vi "Word Example.vi"() -> ()   [LabVIEW 2017]
uses:
  LabVIEW NPOI/MS-Word/MS-Word.lvclass
  C:/Users/Neo/Desktop/Dev_Tools_BR/LabVIEW_NPOI/src/LabVIEW NPOI/Document/Document.lvclass
  LabVIEW NPOI/Document/Document.lvclass/Document.ctl
  LabVIEW NPOI/Document/Get FilePath.vi
  LabVIEW NPOI/Document/Append Table (double).vi
  LabVIEW NPOI/Document/Append Table (string).vi
  LabVIEW NPOI/Document/Read Table As String.vi
  LabVIEW NPOI/Document/Document.lvclass
panel:
  in  "createDocumentBttn":bool
  in  "Text":string="Lorem ipsum dolor sit amet, consectetur adipiscing elit, sed do eiusmod tempor incididunt ut labore et dolore magna aliqua. Adipiscing bibendum est ultricies integer quis auctor elit sed vulputate. Volutpat consequat mauris nunc congue nisi vitae suscipit tellus. Eget arcu dictum varius duis at consectetur lorem donec massa. Morbi enim nunc faucibus a pellentesque sit. Risus ultricies tristique nulla aliquet enim tortor at. Sit amet consectetur adipiscing elit ut aliquam purus sit. Porta lorem mollis aliquam ut porttitor leo a diam. Odio aenean sed adipiscing diam donec adipiscing tristique risus. Nunc eget lorem dolor sed viverra ipsum nunc aliquet. Ultrices gravida dictum fusce ut. Mi eget mauris pharetra et ultrices. Ultrices dui sapien eget mi proin. Duis ut diam quam nulla porttitor massa id neque. Eu lobortis elementum nibh tellus molestie nunc non. Iaculis nunc sed augue lacus viverra. Enim sed faucibus turpis in eu. Quis viverra nibh cras pulvinar mattis. Auctor augue mauris augue neque gravida. Enim ut tellus elementum sagittis vitae."
  in  "addParagraphBttn":bool
  in  "HTML File Path":path
  in  "convertToHtml":bool
  out "Read Table Time":u32
  out "Add Table Time":u32
  in  "addImageBttn":bool
  out "Table Control":string[][](table)
  in  "readTableBttn":bool
  in  "#Columns":i32=100
  in  "#Rows":i32=2
  in  "tableType":enum32{"Strings", "Doubles"}(radio)
  in  "addTableBttn":bool
  out "FilePath":path
  in  "openDocumentBttn":bool
  in  "baseDocumentPath":path caption="Folder Path"
  in  "saveAsDocumentBttn":bool
  in  "saveDocumentBttn":bool
  in  "documentName":string="Book1.xlsx" caption="Name"
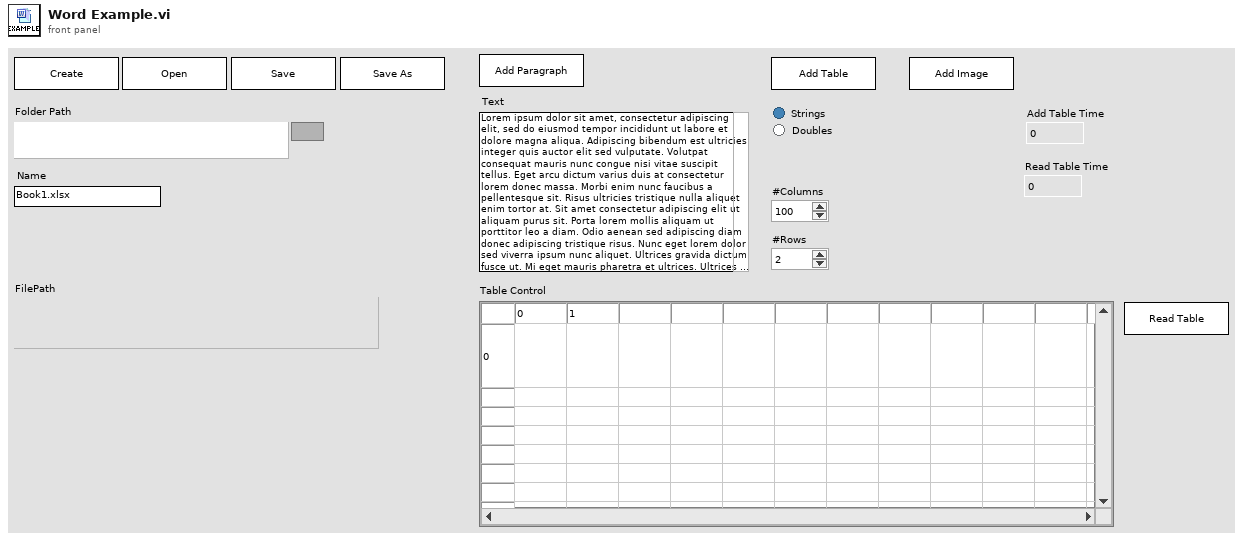
[diagram p1: front panel]
types:
  T1 = cluster{"documentObject":refnum<class "MS-Word.lvclass">, "documentPath":path, "documentName":string, "pageName":string, "styleName":string, "ctlRefs":refnum<vi>[]}
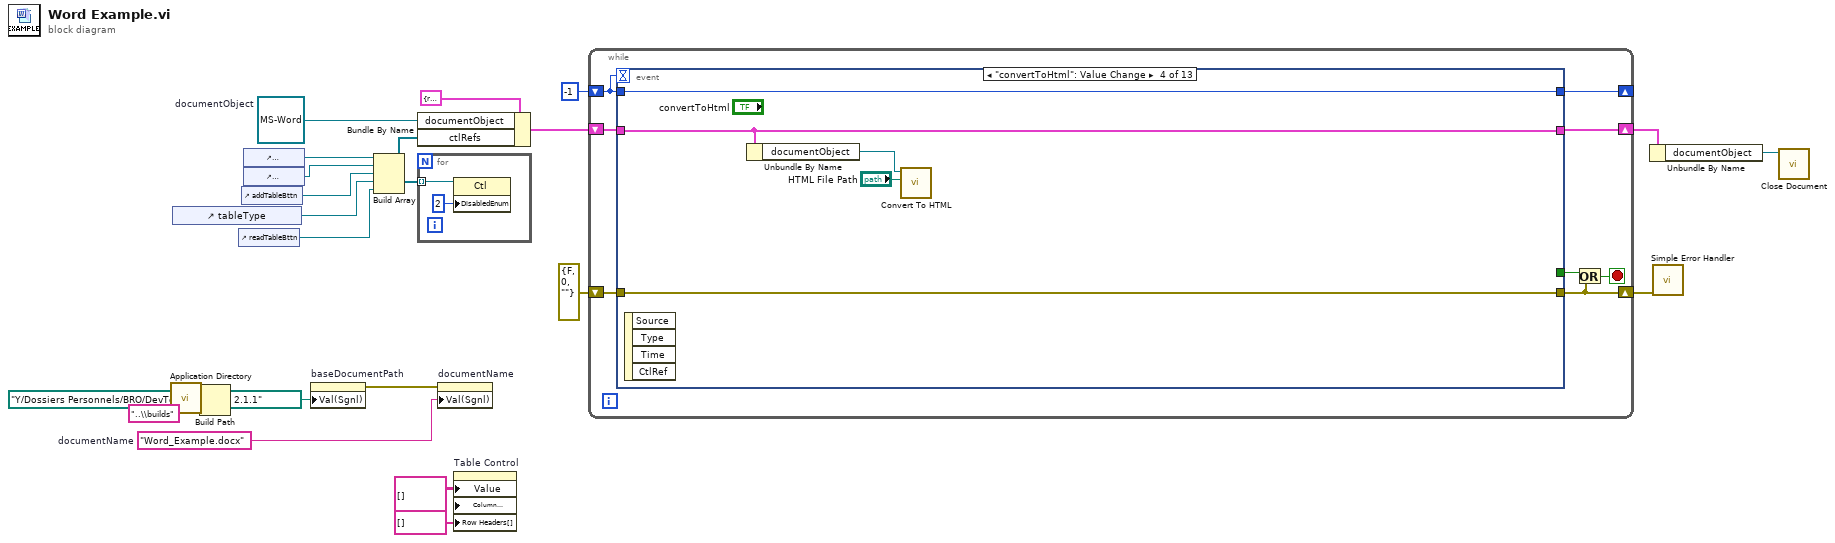
[diagram p0: block diagram]
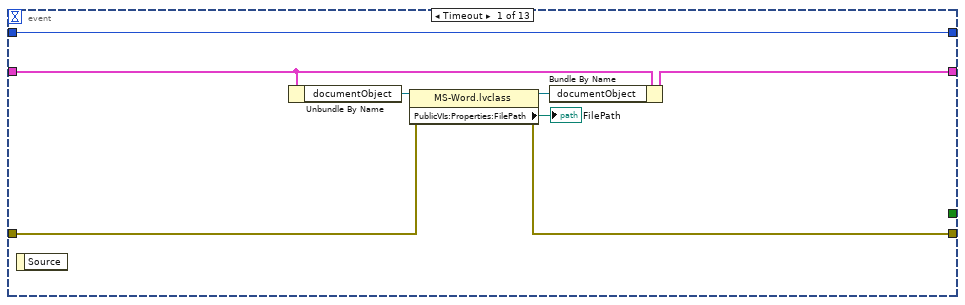
[diagram p2: hidden frame]
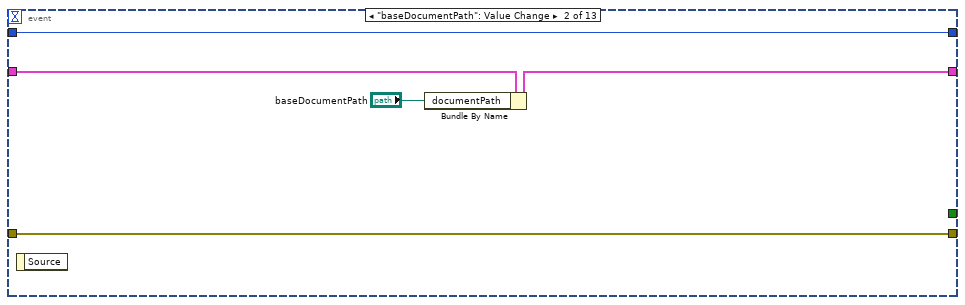
[diagram p3: hidden frame]
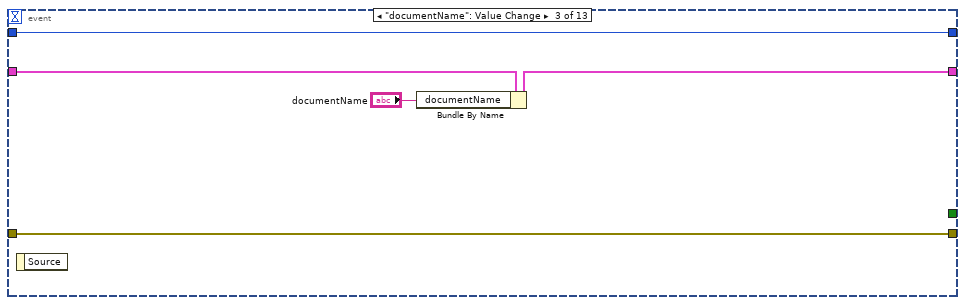
[diagram p4: hidden frame]
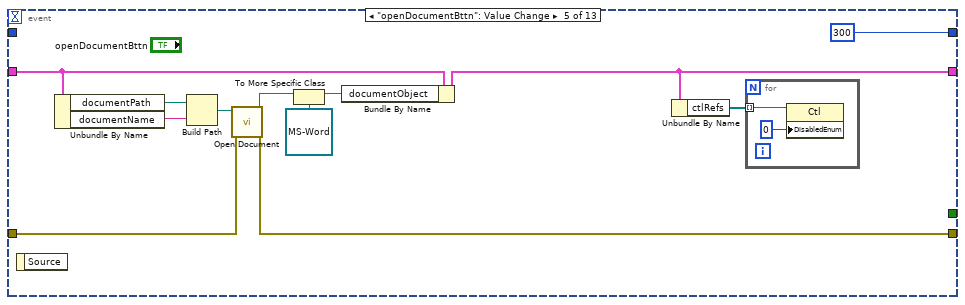
[diagram p5: hidden frame]
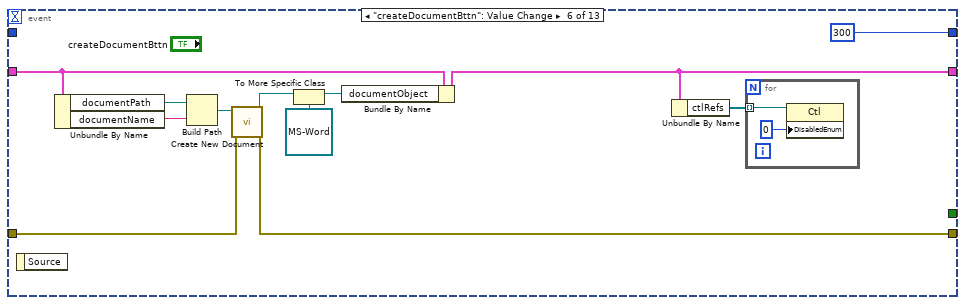
[diagram p6: hidden frame]
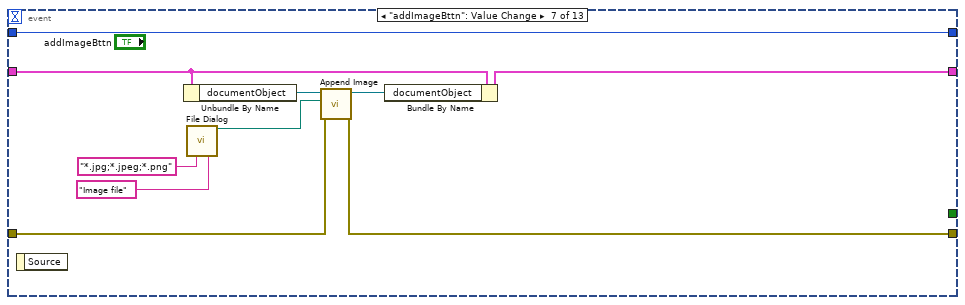
[diagram p7: hidden frame]
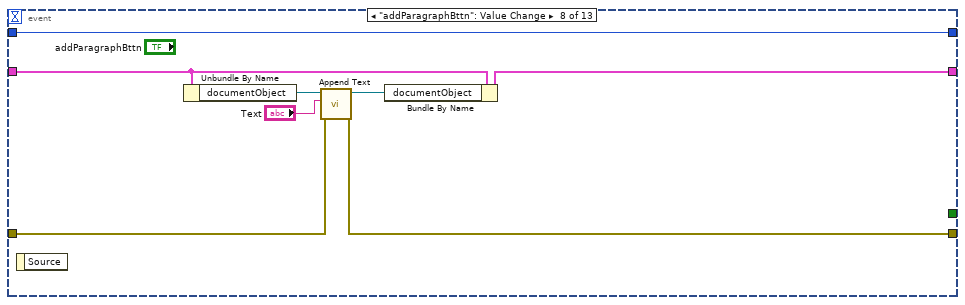
[diagram p8: hidden frame]
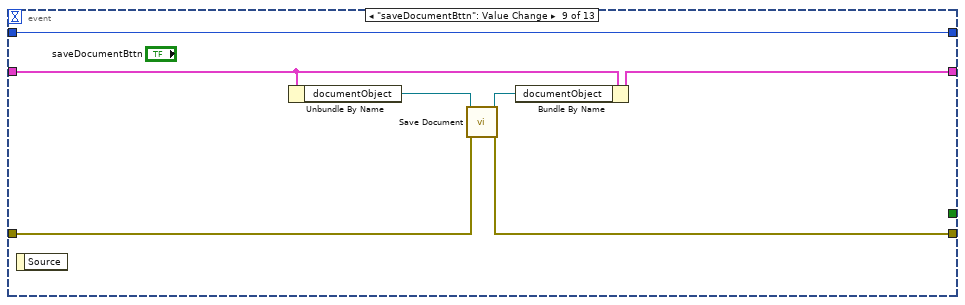
[diagram p9: hidden frame]
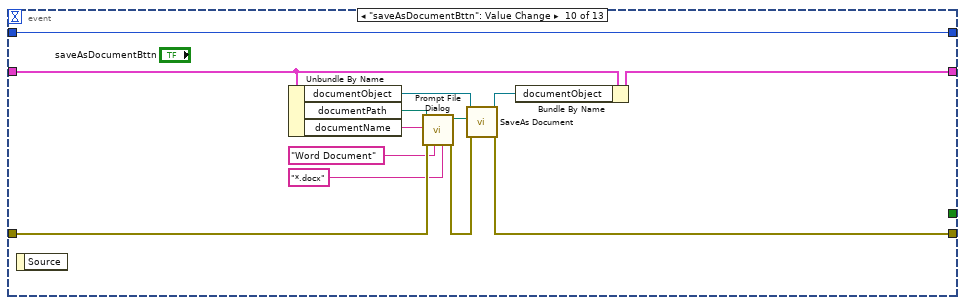
[diagram p10: hidden frame]
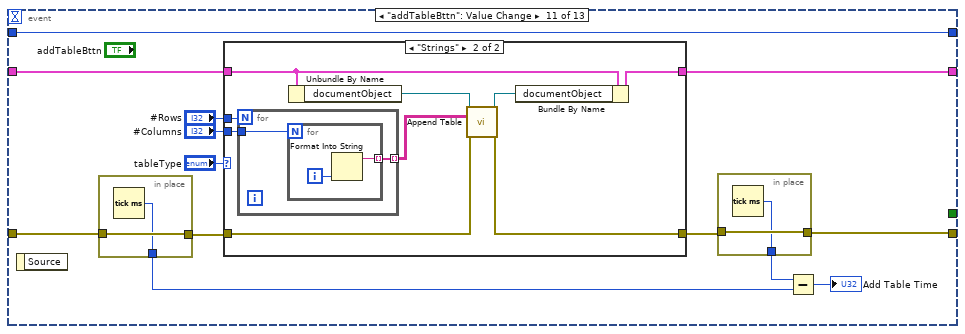
[diagram p11: hidden frame]
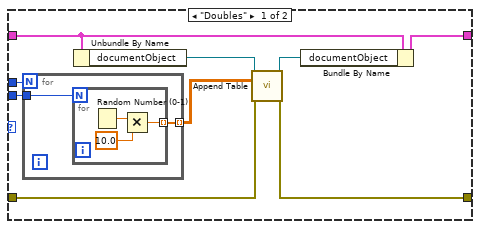
[diagram p12: hidden frame]
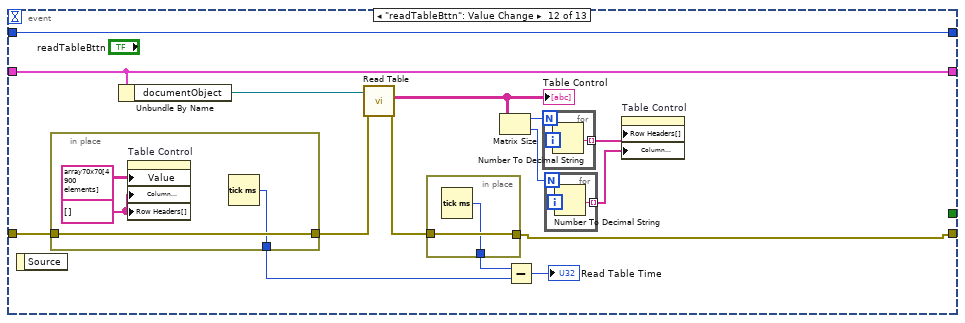
[diagram p13: hidden frame]
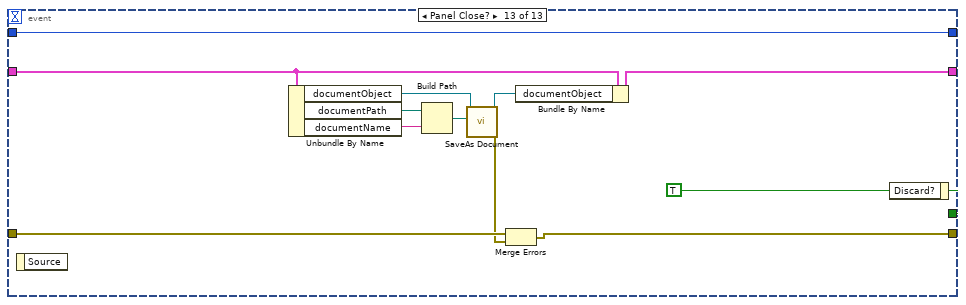
[diagram p14: hidden frame]
diagram:
  w5 = string[] [] ("Row Header Strings[]")
  w10 = "Word_Example.docx"  # documentName
  w14 = refnum<class "MS-Word.lvclass"> refnum  # documentObject
  n1 = call <vilib>:"Application Directory.vi"() -> ("Application Directory"=w4:path)
  n2 = control-ref of="tableType"() -> (w8:refnum<vi>)
  n3 = Build Path(base path=w4, name or relative path="..\\builds") -> ()  [unwired: 1 out]
  n4 = control-ref of="readTableBttn"() -> (w7:refnum<vi>)
  n5 = control-ref of="addTableBttn"() -> (w9:refnum<vi>)
  n6 = control-ref of="saveDocumentBttn"() -> (w13:refnum<vi>)
  n7 = control-ref of="saveAsDocumentBttn"() -> (w12:refnum<vi>)
  n8 = property on="baseDocumentPath" class="Path"("Val(Sgnl)"=path "Y:/Dossiers Personnels/BRO/DevTools_BR/NPOI 2.1.1" ("Value (Signaling)")) -> (error out=w2:errorcluster)  [unwired: 2 in, 1 out]
  n9 = Build Array(w13, w12, w9, w8, w7) -> (w11:refnum<vi>[])
  n10 = Bundle By Name(cluster=T1 {"documentObject"=refnum, "documentPath"=path "", "documentName"="", "pageName"="", "styleName"="Default", "ctlRefs"=[]}, "documentObject"=w14, "ctlRefs"=w11) -> (w21:T1)
  n11 = for {
    tunnel: w11 -> [w23] mode=indexing
    n12 = property class="Ctl"(reference=w23, "DisabledEnum"=u8 2) -> ()  [unwired: 1 in, 2 out]
  }
  n13 = property on="documentName" class="Str"(error in=w2, "Val(Sgnl)"=w10) -> ()  [unwired: 1 in, 2 out]
  n14 = property on="Table Control" class="Tbl (strict)"("Value"=string[][] [] ("Table Control"), "Column Headers[]"=w5, "Row Headers[]"=w5) -> ()  [unwired: 2 in, 2 out]
  n15 = while {
    shift-right: [w30] -> w17
    shift-left: w21 -> [w31]
    shift-right: [w28] -> w20
    shift-left: errorcluster {"status"=FALSE, "code"=0, "source"=""} ("error IO") -> [w29]
    shift-right: [w24] -> _
    shift-left: -1 -> [w25]
    stop <- w26 stop-if-true
    n16 = event shown="[3] \"convertToHtml\": Value Change" {
      selector: _ -> [_ _ _ _ _ _ _ _ _ _ _ _ _]
      dyn-events: _ -> [_ _ _ _ _ _ _ _ _ _ _ _ _]
      timeout: w25 -> [_ _ _ _ _ _ _ _ _ _ _ _ _]
      tunnel: [_ _ _ _ _ _ _ _ _ _ _ _ w194] -> w27
      tunnel: w31 -> [w39 w44 w49 w52 w66 w80 w91 w99 w107 w120 w128 w178 w201]
      tunnel: [w32 w43 w48 w52 w61 w75 w87 w95 w105 w118 w133 w178 w196] -> w30
      tunnel: [w35 w41 w46 w54 w55 w69 w88 w96 w103 w116 w124 w168 w192] -> w28
      tunnel: w29 -> [w36 w41 w46 w54 w63 w77 w89 w97 w102 w114 w127 w171 w193]
      tunnel: w25 -> [w33 w40 w45 w53 _ _ w92 w100 w101 w108 w132 w179 w190]
      tunnel: [w33 w40 w45 w53 300 300 w92 w100 w101 w108 w132 w179 w190] -> w24
      event Timeout {
        n17 = event-data() -> ()  [unwired: 1 in, 1 out]
        n18 = Unbundle By Name(w39) -> ("documentObject"=w38:refnum<class "MS-Word.lvclass">)
        n19 = property class="MS-Word.lvclass"(reference=w38, error in=w36) -> (reference out=w37:refnum<class "MS-Word.lvclass">, error out=w35:errorcluster, "PublicVIs:Properties:FilePath"=→"FilePath":path)
        n20 = Bundle By Name(cluster=w39, "documentObject"=w37) -> (w32:T1)
      }
      event "baseDocumentPath": Value Change {
        n21 = event-data() -> ()  [unwired: 1 in, 1 out]
        n22 = Bundle By Name(cluster=w44, "documentPath"="baseDocumentPath") -> (w43:T1)
      }
      event "documentName": Value Change {
        n23 = event-data() -> ()  [unwired: 1 in, 1 out]
        n24 = Bundle By Name(cluster=w49, "documentName"="documentName") -> (w48:T1)
      }
      event "convertToHtml": Value Change {
        n25 = event-data() -> ()  [unwired: 1 in, 4 out]
        n26 = Unbundle By Name(w52) -> ("documentObject"=w51:refnum<class "MS-Word.lvclass">)
        n27 = call "Convert To HTML.vi"("HTML File Path"="HTML File Path", "Document in"=w51) -> ()  [unwired: 8 in, 2 out]
      }
      event "openDocumentBttn": Value Change {
        n28 = event-data() -> ()  [unwired: 1 in, 1 out]
        n29 = Unbundle By Name(w66) -> ("documentPath"=w65:path, "documentName"=w64:string)
        n30 = Build Path(base path=w65, name or relative path=w64) -> (appended path=w59:path)
        n31 = call "Open Document.vi"("error in (no error)"=w63, "File Path"=w59) -> ("error out"=w55:errorcluster, "Document out"=w57:refnum<class "Document.lvclass">)  [unwired: 8 in]
        n32 = To More Specific Class(target class=refnum<class "MS-Word.lvclass"> refnum ("workbookObject"), reference=w57) -> (specific class reference=w56:refnum<class "MS-Word.lvclass">)  [unwired: 1 in, 1 out]
        n33 = Bundle By Name(cluster=w66, "documentObject"=w56) -> (w61:T1)
        n34 = Unbundle By Name(w61) -> ("ctlRefs"=w60:refnum<vi>[])
        n35 = for {
          tunnel: w60 -> [w68] mode=indexing
          n36 = property class="Ctl"(reference=w68, "DisabledEnum"=u8 0) -> ()  [unwired: 1 in, 2 out]
        }
      }
      event "createDocumentBttn": Value Change {
        n37 = event-data() -> ()  [unwired: 1 in, 1 out]
        n38 = Unbundle By Name(w80) -> ("documentPath"=w79:path, "documentName"=w78:string)
        n39 = Build Path(base path=w79, name or relative path=w78) -> (appended path=w73:path)
        n40 = call "Create New Document.vi"("error in (no error)"=w77, "File Path"=w73) -> ("error out"=w69:errorcluster, "Document out"=w71:refnum<class "Document.lvclass">)  [unwired: 8 in]
        n41 = To More Specific Class(target class=refnum<class "MS-Word.lvclass"> refnum ("workbookObject"), reference=w71) -> (specific class reference=w70:refnum<class "MS-Word.lvclass">)  [unwired: 1 in, 1 out]
        n42 = Bundle By Name(cluster=w80, "documentObject"=w70) -> (w75:T1)
        n43 = Unbundle By Name(w75) -> ("ctlRefs"=w74:refnum<vi>[])
        n44 = for {
          tunnel: w74 -> [w82] mode=indexing
          n45 = property class="Ctl"(reference=w82, "DisabledEnum"=u8 0) -> ()  [unwired: 1 in, 2 out]
        }
      }
      event "addImageBttn": Value Change {
        n46 = event-data() -> ()  [unwired: 1 in, 1 out]
        n47 = Unbundle By Name(w91) -> ("documentObject"=w90:refnum<class "MS-Word.lvclass">)
        n48 = call "File Dialog"("pattern (all files)"="*.jpg;*.jpeg;*.png", "pattern label"="Image file") -> ("selected path"=w85:path)  [unwired: 10 in, 3 out]
        n49 = call "Append Image.vi"("error in (no error)"=w89, "Image File Path"=w85, "Document in"=w90) -> ("error out"=w88:errorcluster, "Document out"=w86:refnum<class "MS-Word.lvclass">)  [unwired: 7 in]
        n50 = Bundle By Name(cluster=w91, "documentObject"=w86) -> (w87:T1)
      }
      event "addParagraphBttn": Value Change {
        n51 = event-data() -> ()  [unwired: 1 in, 1 out]
        n52 = Unbundle By Name(w99) -> ("documentObject"=w98:refnum<class "MS-Word.lvclass">)
        n53 = call "Append Text.vi"("error in (no error)"=w97, "Text"="Text", "Document in"=w98) -> ("error out"=w96:errorcluster, "Document out"=w94:refnum<class "MS-Word.lvclass">)  [unwired: 7 in]
        n54 = Bundle By Name(cluster=w99, "documentObject"=w94) -> (w95:T1)
      }
      event "saveDocumentBttn": Value Change {
        n55 = event-data() -> ()  [unwired: 1 in, 1 out]
        n56 = Unbundle By Name(w107) -> ("documentObject"=w106:refnum<class "MS-Word.lvclass">)
        n57 = call "Save Document.vi"("error in (no error)"=w102, "Document in"=w106) -> ("error out"=w103:errorcluster, "Document out"=w104:refnum<class "MS-Word.lvclass">)  [unwired: 8 in]
        n58 = Bundle By Name(cluster=w107, "documentObject"=w104) -> (w105:T1)
      }
      event "saveAsDocumentBttn": Value Change {
        n59 = event-data() -> ()  [unwired: 1 in, 1 out]
        n60 = Unbundle By Name(w120) -> ("documentObject"=w119:refnum<class "MS-Word.lvclass">, "documentPath"=w110:path, "documentName"=w109:string)
        n61 = call "Prompt File Dialog.vi"("pattern (all files)"="*.docx", "pattern label"="Word Document", "error in"=w114, "default name"=w109, "File Path"=w110) -> ("error out"=w113:errorcluster, "selected path"=w115:path)  [unwired: 5 in]
        n62 = call "SaveAs Document.vi"("error in (no error)"=w113, "File Path"=w115, "Document in"=w119) -> ("error out"=w116:errorcluster, "Document out"=w117:refnum<class "MS-Word.lvclass">)  [unwired: 7 in]
        n63 = Bundle By Name(cluster=w120, "documentObject"=w117) -> (w118:T1)
      }
      event "addTableBttn": Value Change {
        n64 = event-data() -> ()  [unwired: 1 in, 1 out]
        n65 = in-place {
          in-place-border: w127 -> [w137]
          in-place-border: [w137] -> w126
          in-place-border: [w136] -> w122
          n66 = Tick Count (ms)() -> (millisecond timer value=w136:u32)
        }
        n67 = case shown="\"Strings\"" "tableType" {
          tunnel: w128 -> [w146 w160]
          tunnel: [w144 w158] -> w133
          tunnel: [w142 w156] -> w125
          tunnel: w126 -> [w141 w155]
          tunnel: "#Columns" -> [w138 w153]
          tunnel: "#Rows" -> [w139 w152]
          frame "Doubles" {
            n68 = for {
              N: w139 -> [_]
              tunnel: [w148] -> w140 mode=indexing
              tunnel: w138 -> [w147]
              n69 = for {
                N: w147 -> [_]
                tunnel: [w150] -> w148 mode=indexing
                n70 = Random Number (0-1)() -> (number: 0 to 1=w151:dbl)
                n71 = Multiply(x=w151, y=10.0) -> (x*y=w150:dbl)
              }
            }
            n72 = Unbundle By Name(w146) -> ("documentObject"=w145:refnum<class "MS-Word.lvclass">)
            n73 = call-poly "Append Table.vi"("Document in"=w145, "Table"=w140, "error in (no error)"=w141) -> ("Document out"=w143:refnum<class "MS-Word.lvclass">, "error out"=w142:errorcluster)  [unwired: 11 in]
            n74 = Bundle By Name(cluster=w146, "documentObject"=w143) -> (w144:T1)
          }
          frame "Strings" {
            n75 = for {
              N: w152 -> [_]
              tunnel: [w162] -> w154 mode=indexing
              tunnel: w153 -> [w161]
              n76 = for {
                N: w161 -> [_]
                tunnel: [w163] -> w162 mode=indexing
                i -> [w164]
                n77 = Format Into String(w164) -> (resulting string=w163:string)  [unwired: 3 in, 1 out]
              }
            }
            n78 = Unbundle By Name(w160) -> ("documentObject"=w159:refnum<class "MS-Word.lvclass">)
            n79 = call-poly "Append Table.vi"("Document in"=w159, "Table"=w154, "error in (no error)"=w155) -> ("Document out"=w157:refnum<class "MS-Word.lvclass">, "error out"=w156:errorcluster)  [unwired: 11 in]
            n80 = Bundle By Name(cluster=w160, "documentObject"=w157) -> (w158:T1)
          }
        }
        n81 = in-place {
          in-place-border: w125 -> [w135]
          in-place-border: [w135] -> w124
          in-place-border: [w134] -> w123
          n82 = Tick Count (ms)() -> (millisecond timer value=w134:u32)
        }
        n83 = Subtract(x=w123, y=w122) -> (x-y=→"Add Table Time":u32)
      }
      event "readTableBttn": Value Change {
        n84 = event-data() -> ()  [unwired: 1 in, 1 out]
        n85 = in-place {
          in-place-border: w171 -> [w183]
          in-place-border: [w183] -> w170
          in-place-border: [w182] -> w166
          w185 = string[] [] ("Row Header Strings[]")
          n86 = property on="Table Control" class="Tbl (strict)"("Value"=string[][] array70x70[4900 elements] ("Table Control"), "Column Headers[]"=w185, "Row Headers[]"=w185) -> ()  [unwired: 2 in, 2 out]
          n87 = Tick Count (ms)() -> (millisecond timer value=w182:u32)
        }
        n88 = Unbundle By Name(w178) -> ("documentObject"=w177:refnum<class "MS-Word.lvclass">)
        n89 = call-poly "Read Table.vi"("error in (no error)"=w170, "Document in"=w177) -> ("error out"=w169:errorcluster, "Table As String"=w176:string[][])  [unwired: 7 in, 1 out]
        "Table Control" <- w176
        n90 = in-place {
          in-place-border: w169 -> [w181]
          in-place-border: [w181] -> w168
          in-place-border: [w180] -> w167
          n91 = Tick Count (ms)() -> (millisecond timer value=w180:u32)
        }
        n92 = Matrix Size(0:w176) -> (1:w175:i32, 2:w173:i32)
        n93 = Subtract(x=w167, y=w166) -> (x-y=→"Read Table Time":u32)
        n94 = for {
          N: w175 -> [_]
          tunnel: [w188] -> w174 mode=indexing
          i -> [w189]
          n95 = Number To Decimal String(number=w189) -> (decimal integer string=w188:string)  [unwired: 1 in]
        }
        n96 = for {
          N: w173 -> [_]
          tunnel: [w186] -> w172 mode=indexing
          i -> [w187]
          n97 = Number To Decimal String(number=w187) -> (decimal integer string=w186:string)  [unwired: 1 in]
        }
        n98 = property on="Table Control" class="Tbl (strict)"("Row Headers[]"=w174, "Column Headers[]"=w172) -> ()  [unwired: 2 in, 2 out]
      }
      event Panel Close? {
        w194 = TRUE ("Discard?")
        n99 = event-data() -> ()  [unwired: 1 in, 1 out]
        n100 = Unbundle By Name(w201) -> ("documentObject"=w198:refnum<class "MS-Word.lvclass">, "documentPath"=w200:path, "documentName"=w199:string)
        n101 = Build Path(base path=w200, name or relative path=w199) -> (appended path=w197:path)
        n102 = call "SaveAs Document.vi"("File Path"=w197, "Document in"=w198) -> ("error out"=w191:errorcluster, "Document out"=w195:refnum<class "MS-Word.lvclass">)  [unwired: 8 in]
        n103 = Merge Errors(w193, w191) -> (w192:errorcluster)
        n104 = Bundle By Name(cluster=w201, "documentObject"=w195) -> (w196:T1)
        n105 = event-data("Discard?"=w194) -> ()  [unwired: 1 in, 1 out]
      }
    }
    n106 = Or(x=w27, y=w28) -> (x .or. y?=w26:bool)
  }
  n107 = Unbundle By Name(w17) -> ("documentObject"=w16:refnum<class "MS-Word.lvclass">)
  n108 = call <vilib>:"Simple Error Handler.vi"("error in (no error)"=w20) -> ()  [unwired: 4 in, 5 out]
  n109 = call "Close Document.vi"("Document in"=w16) -> ()  [unwired: 10 in, 1 out]
